vi "WriteDefaultSubpanel.vi"(8 "error in (no error)":errorcluster, 10 "SMO.UI.Embedded":refnum<class "Embedded UI.lvclass">, 11 "SMO.UI.MAUI in":refnum<class "MAUI.lvclass">) -> (0 "error out":errorcluster, 3 "SMO.UI.MAUI out":refnum<class "MAUI.lvclass">)   [LabVIEW 2019, in "MAUI.lvclass"]
uses:
  MAUI.lvclass
  <userlib>/LevyLab/Embedded UI/SMO.UI.Embedded/Embedded UI.lvclass
  Typedefs/DefaultSubpanel.ctl
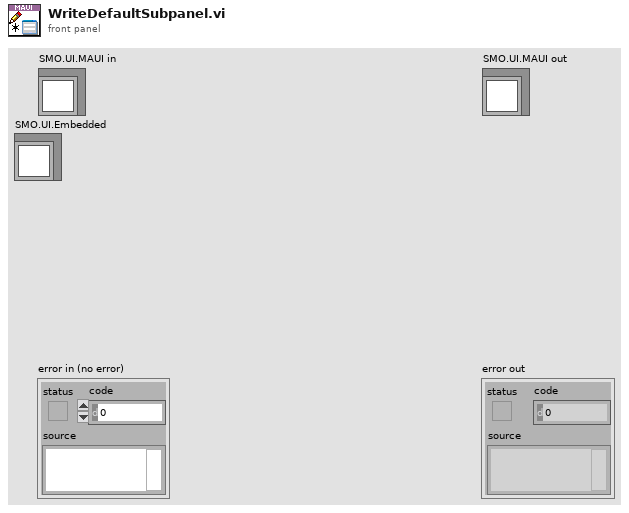
[diagram p1: front panel]
types:
  T1 = typedef "MAUI.lvclass/DefaultSubpanel.ctl" = cluster{"SMO.UI.Embedded":refnum<class "Embedded UI.lvclass">}
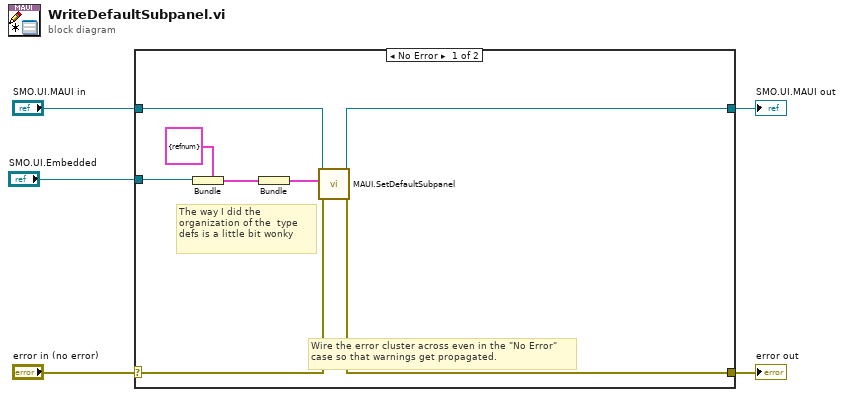
[diagram p0: block diagram]
diagram:
  n1 = case shown="No Error" "error in (no error)" {
    selector: "error in (no error)" -> [w7 w15]
    tunnel: [w6 w15] -> w4
    tunnel: [w9 w14] -> w2
    tunnel: "SMO.UI.MAUI in" -> [w8 w14]
    tunnel: "SMO.UI.Embedded" -> [w13 _]
    frame No Error {
      # "The way I did the organization of the  type defs is a little bit wonky"
      # "Wire the error cluster across even in the \"No Error\"\ncase so that warnings get propagated."
      n2 = Bundle(cluster=T1 {"SMO.UI.Embedded"=refnum} ("Default Subpanel"), "SMO.UI.Embedded"=w13) -> (w11:T1)
      n3 = Bundle("Default Subpanel"=w11) -> (w10:cluster{"Default Subpanel":T1})  [unwired: 1 in]
      n4 = call "MAUI.SetDefaultSubpanel.vi"("error in (no error)"=w7, "SetDefaultSubpanel"=w10, "SMO.UI.MAUI"=w8) -> ("error out"=w6:errorcluster, "SMO.UI.MAUI out"=w9:refnum<class "MAUI.lvclass">)  [unwired: 7 in]
    }
    frame Error {
    }
  }
  "error out" <- w4
  "SMO.UI.MAUI out" <- w2
